vi "Enable Disable.vi"(8 "error in (no error)":errorcluster, 11 "Node Ptr":T1 format="%.0x") -> (0 "error out":errorcluster)   [LabVIEW 2020, in "Modbus Master System Explorer.lvlib"]
uses:
  Modbus Master System Explorer.lvlib
  <vilib>/NI VeriStand/Custom Device API/Custom Device Item Ref.ctl
  Shared/Constants.vi
  <vilib>/NI VeriStand/Custom Device API/Custom Device API.lvlib
  Shared/Modbus Master Shared.lvlib
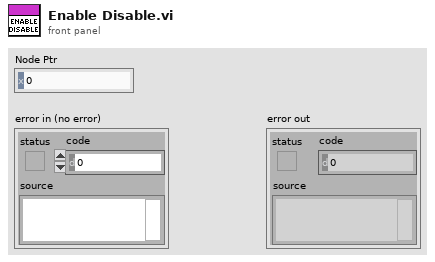
[diagram p1: front panel]
types:
  T1 = typedef "Custom Device API.lvlib/Custom Device Item Ref.ctl" = u64
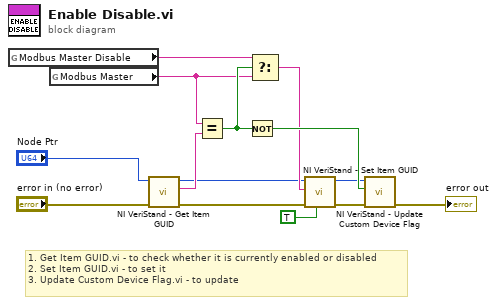
[diagram p0: block diagram]
diagram:
  # "1. Get Item GUID.vi - to check whether it is currently enabled or disabled\n2. Set Item GUID.vi - to set it\n3. Update Custom Device Flag.vi - to update"
  n1 = global read "Constants.vi" "Modbus Master Disable"() -> (w1:string)
  n2 = global read "Constants.vi" "Modbus Master"() -> (w2:string)
  n3 = call <vilib>:"NI VeriStand - Get Item GUID.vi"("error in (no error)"="error in (no error)", "Item Ref in"="Node Ptr") -> ("error out"=w5:errorcluster, "GUID"=w10:string, "Item Ref out"=w6:T1)  [unwired: 7 in]
  n4 = Equal?(x=w2, y=w10) -> (x = y?=w11:bool)
  n5 = Not(x=w11) -> (.not. x?=w13:bool)
  n6 = Select(t=w1, s=w11, f=w2) -> (s? t:f=w12:string)
  n7 = call <vilib>:"NI VeriStand - Set Item GUID.vi"("Refresh System Explorer Tree? (F)"=TRUE, "error in (no error)"=w5, "GUID"=w12, "Item Ref in"=w6) -> ("error out"=w7:errorcluster, "Item Ref out"=w8:T1)  [unwired: 6 in]
  n8 = call <vilib>:"NI VeriStand - Update Custom Device Flag.vi"("error in (no error)"=w7, "Is Custom Device Active?"=w13, "Device Ref in"=w8) -> ("error out"=→"error out":errorcluster)  [unwired: 7 in, 1 out]
